vi "send16bit UINT Volume Data To Sink.vi"(0 "pSinkId":i32, 1 "pWidthInVoxels":i32, 2 "pDepthInVoxels":i32, 5 "pChannelId":i32, 7 "pBufferAddress":i16, 9 "pBufferLength":i64, 11 "error in (no error)":errorcluster, 12 "pHeightInVoxels":i32) -> (4 "function return":i32, 8 "pBufferAddress out":i16, 15 "error out":errorcluster)   [LabVIEW 2012, in "clearvolume.lvlib"]
doc: "__declspec(dllexport) long __cdecl send16bitUINTVolumeDataToSink( long pSinkId,\n long pChannelId,\n short *pBufferAddress,\n __int64 pBufferLength, \n long pWidthInVoxels,\n long pHeightInVoxels,\n long pDepthInVoxels);"
uses:
  clearvolume.lvlib
  clearvolume.dll
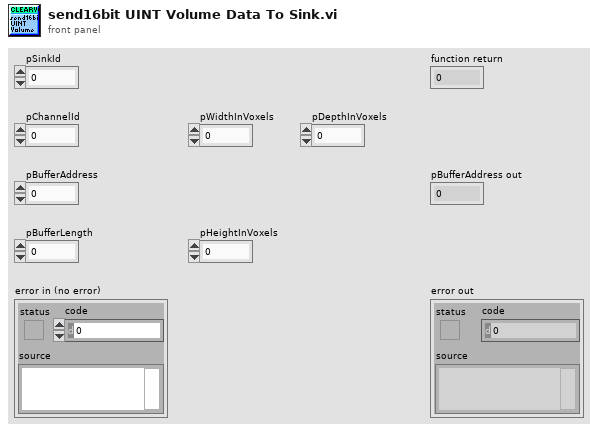
[diagram p1: front panel]
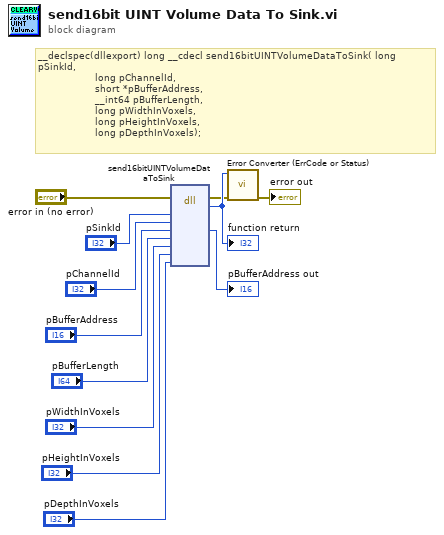
[diagram p0: block diagram]
diagram:
  # "__declspec(dllexport) long __cdecl send16bitUINTVolumeDataToSink( long pSinkId,\n\t\t\t\t\t\t\t\t\t\t\t\t\t\t\t\t\t\t\tlong pChannelId,\n\t\t\t\t\t\t\t\t\t\t\t\t\t\t\t\t\t\t\tshort *pBufferAddress,\n\t\t\t\t\t\t\t\t\t\t\t\t\t\t\t\t\t\t\t__int64 pBufferLength,\t\t\t\t\t\t\t\t\t\t\t\t\t\t\t\t\t\t\t\n\t\t\t\t\t\t\t\t\t\t\t\t\t\t\t\t\t\t\tlong pWidthInVoxels,\n\t\t\t\t\t\t\t\t\t\t\t\t\t\t\t\t\t\t\tlong pHeightInVoxels,\n\t\t\t\t\t\t\t\t\t\t\t\t\t\t\t\t\t\t\tlong pDepthInVoxels);"
  n1 = dll-call lib="C:/Users/myerslab/workspace/Libraries/CV/clearvolume/src/labview/clearvolume/clearvolume.*" fn="send16bitUINTVolumeDataToSink"(error in="error in (no error)", "pSinkId"="pSinkId", "pChannelId"="pChannelId", "pBufferAddress"="pBufferAddress", "pBufferLength"="pBufferLength", "pWidthInVoxels"="pWidthInVoxels", "pHeightInVoxels"="pHeightInVoxels", "pDepthInVoxels"="pDepthInVoxels") -> (error out=w2:errorcluster, w12:i32, "pBufferAddress"=→"pBufferAddress out":i16)  [unwired: 8 in, 1 out]
  "function return" <- w12
  n2 = call "Error Converter (ErrCode or Status).vi"("error in (no error)"=w2, "error code"=w12) -> ("error out"=→"error out":errorcluster)  [unwired: 9 in]
